vi "String_operations.vi"() -> ()   [LabVIEW 2019]
panel:
  out "trimmed string":string
  out "length 3":i32
  in  "String 6":string="String with white spaces trimmed"
  out "length 2":i32
  out "substring":string
  in  "String 5":string="Subset of a given string"
  out "length":i32
  in  "String 4":string
  in  "string 3":string="Concatenation"
  in  "string 2":string="String"
  in  "string 1":string="This is"
  out "concatenated string":string
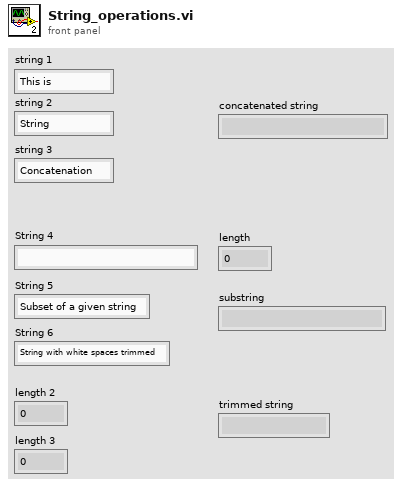
[diagram p1: front panel]
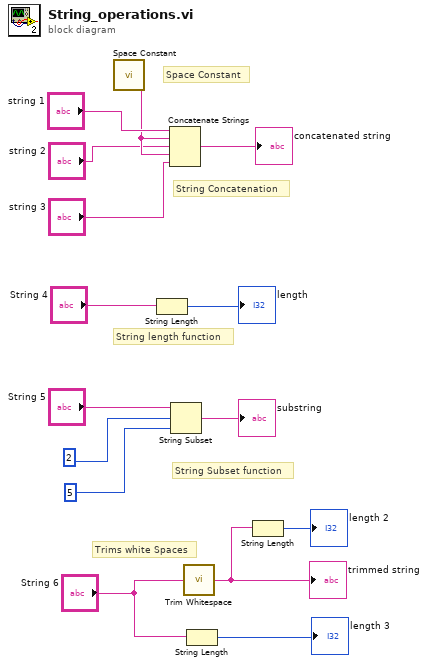
[diagram p0: block diagram]
diagram:
  # "Trims white Spaces"
  # "String Subset function"
  # "String length function"
  # "String Concatenation"
  # "Space Constant"
  n1 = call <vilib>:"Space Constant.vi"() -> ("String"=w13:string)
  n2 = String Length(string="String 4") -> (length=→"length":i32)
  n3 = Concatenate Strings("string 1", w13, "string 2", w13, "string 3") -> (→"concatenated string":string)
  n4 = String Subset(string="String 5", offset (0)=2, length (rest)=5) -> (substring=→"substring":string)
  n5 = call <vilib>:"Trim Whitespace.vi"("string"="String 6") -> ("trimmed string"=w1:string)  [unwired: 1 in]
  "trimmed string" <- w1
  n6 = String Length(string="String 6") -> (length=→"length 3":i32)
  n7 = String Length(string=w1) -> (length=→"length 2":i32)
